vi "push_boolean_array.vi"(8 "error in (no error)":errorcluster, 10 "value":bool[](array[boolean]), 11 "Lua in":refnum<class "Lua.lvclass">) -> (0 "error out":errorcluster, 3 "Lua out":refnum<class "Lua.lvclass">)   [LabVIEW 2020, in "Lua for LabVIEW.lvlib" / "Lua.lvclass"]
doc: "Push a numeric array to the Lua stack (creates a lua table)."
uses:
  Lua.lvclass
  Lua.lvclass/Lua.ctl
  lib/lua.dll/lua.dll.lvlib
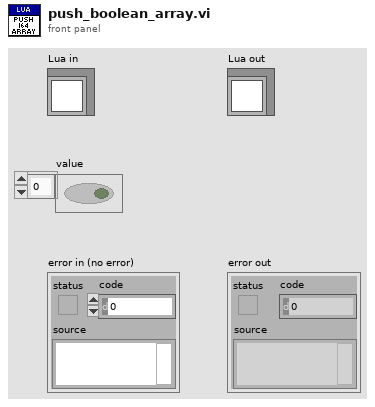
[diagram p1: front panel]
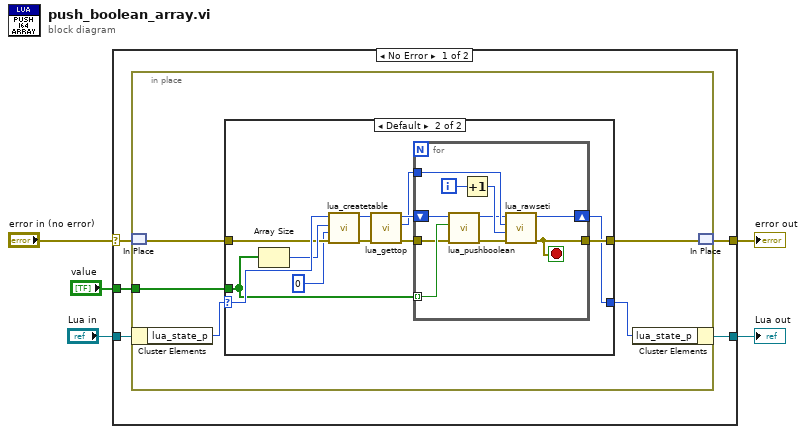
[diagram p0: block diagram]
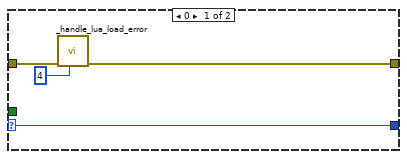
[diagram p2: hidden frame]
diagram:
  n1 = case shown="No Error" "error in (no error)" {
    selector: "error in (no error)" -> [w7 w43]
    tunnel: [w8 w43] -> w4
    tunnel: [w9 w42] -> w2
    tunnel: "Lua in" -> [w10 w42]
    tunnel: "value" -> [w6 _]
    frame No Error {
      n2 = in-place {
        in-place-border: w6 -> [w12]
        n3 = in-place-match #1(w7) -> (w14:errorcluster)
        n4 = in-place-cluster #2(w10) -> ("lua_state_p"=w15:u64)
        n5 = case shown="Default" w15 {
          selector: w15 -> [w19 w31]
          tunnel: [w19 w21] -> w11
          tunnel: w14 -> [w16 w29]
          tunnel: [w17 w26] -> w13
          tunnel: w12 -> [_ w27]
          frame 0 {
            n6 = call "_handle_lua_load_error.vi"("lua_load errcode"=4, "error in (no error)"=w16) -> ("error out"=w17:errorcluster)  [unwired: 9 in]
          }
          frame Default {
            n7 = Array Size(array=w27) -> (size(s)=w30:i32)
            n8 = call "lua_createtable.vi"("error in (no error)"=w29, "nrec"=0, "narr"=w30, "lua_state_p"=w31) -> ("error out"=w25:errorcluster, "lua_state_p out"=w24:u64)  [unwired: 6 in]
            n9 = call "lua_gettop.vi"("error in (no error)"=w25, "lua_state_p"=w24) -> ("error out"=w23:errorcluster, "index"=w20:i32, "lua_state_p out"=w22:u64)  [unwired: 7 in]
            n10 = for {
              shift-right: [w35] -> w21
              shift-left: w22 -> [w39]
              tunnel: w23 -> [w38]
              tunnel: w27 -> [w41] mode=indexing
              tunnel: [w36] -> w26
              tunnel: w20 -> [w34]
              i -> [w40]
              stop <- w36 stop-if-true
              n11 = call "lua_pushboolean.vi"("error in (no error)"=w38, "Boolean"=w41, "lua_state_p"=w39) -> ("error out"=w32:errorcluster, "lua_state_p out"=w33:u64)  [unwired: 7 in]
              n12 = Increment(x=w40) -> (x+1=w37:i32)
              n13 = call "lua_rawseti.vi"("error in (no error)"=w32, "n"=w37, "index"=w34, "lua_state_p"=w33) -> ("error out"=w36:errorcluster, "lua_state_p out"=w35:u64)  [unwired: 6 in]
            }
          }
        }
        n14 = in-place-cluster #2("lua_state_p"=w11) -> (w9:refnum<class "Lua.lvclass">)
        n15 = in-place-match #1(w13) -> (w8:errorcluster)
      }
    }
    frame Error {
    }
  }
  "error out" <- w4
  "Lua out" <- w2
